vi "Configure Measurement Characteristics (Frequency-Power).vi"(0 "VISA resource name":refnum<visa-resource-name>, 1 "Trace 1 Format Settings":T2={"Frequency Format (1: Hz)"=enum."Hz", "Sensitivity Aperture (1 %)"=1.0, "Frequency Reference (0 Hz)"=0.0} {"Frequency Reference (0 Hz)" format="%^#_9g"; "Sensitivity Aperture (1 %)" format="%^#_9g"}, 5 "Frequency Band (1: High)":u16(ring)=1 items=["Low (10E6 to 1.5E9 Hz)", "High (250E6 to 7E9 Hz)", "Band 3 (3E9 to 10E9 Hz)", "Band 4 (9E9 to 26.5E9 Hz)"], 7 "Enable Carrier Search (Disable)":bool, 9 "Manual Nominal Frequency (3E9 Hz)":dbl=3000000000.0 format="%^#_9g", 11 "error in (no error)":errorcluster, 12 "Trace 4 Format Settings":T1={"Frequency Format (2: Hz/V)"=enum."Hz/V", "Sensitivity Aperture (1 %)"=1.0, "Frequency Reference (0 Hz)"=0.0} {"Frequency Reference (0 Hz)" format="%^#_9g"; "Sensitivity Aperture (1 %)" format="%^#_9g"}) -> (4 "VISA resource name out":refnum<visa-resource-name>, 15 "error out":errorcluster)   [LabVIEW 2011, in "Agilent E5052X.lvlib"]
doc: "Configures initial settings for Frequency/Power measurement. \n\n<b>Note: </b>\n\n1) This VI must be called first before calling \"Configure Measurement(Freq-Power)\" VI.\n\n2) Only Trace 1 and 4 format settings can be changed. Trace 2 and 3 are constantly set for Power and Current respectively."
uses:
  Agilent E5052X.lvlib
panel:
  # "Input Frequency Setting"
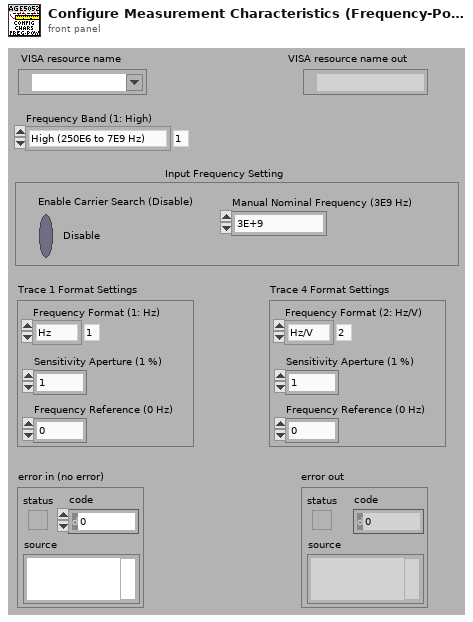
[diagram p1: front panel]
types:
  T1 = cluster{"Frequency Format (2: Hz/V)":enum16{"DHz", "Hz", "Hz/V", "Percent", "ppm"}, "Sensitivity Aperture (1 %)":dbl, "Frequency Reference (0 Hz)":dbl}
  T2 = cluster{"Frequency Format (1: Hz)":enum16{"DHz", "Hz", "Hz/V", "Percent", "ppm"}, "Sensitivity Aperture (1 %)":dbl, "Frequency Reference (0 Hz)":dbl}
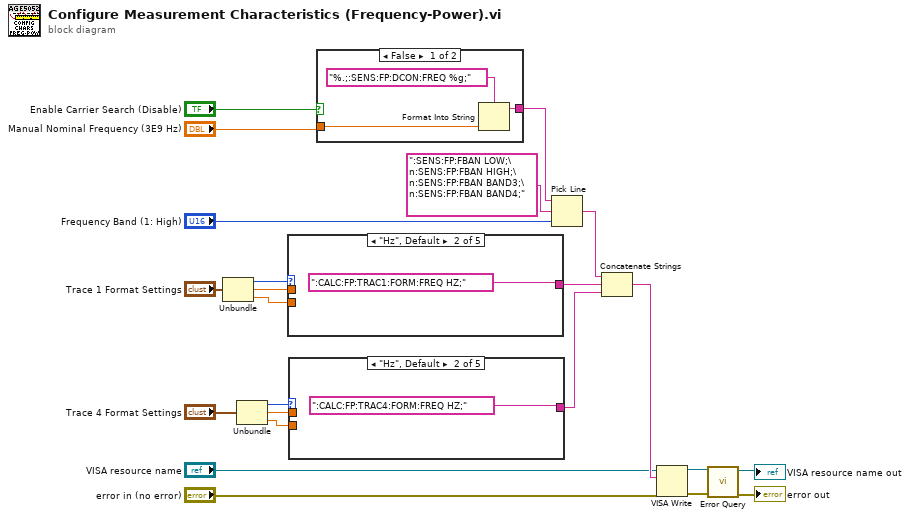
[diagram p0: block diagram]
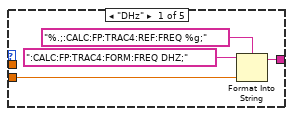
[diagram p2: hidden frame]
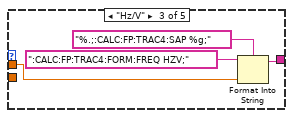
[diagram p3: hidden frame]
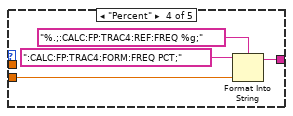
[diagram p4: hidden frame]
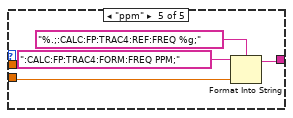
[diagram p5: hidden frame]
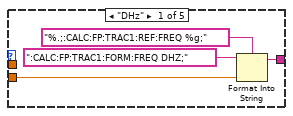
[diagram p6: hidden frame]
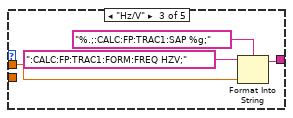
[diagram p7: hidden frame]
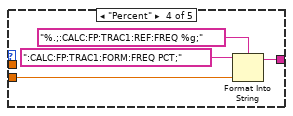
[diagram p8: hidden frame]
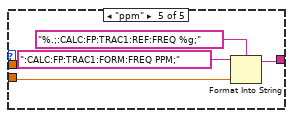
[diagram p9: hidden frame]
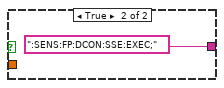
[diagram p10: hidden frame]
diagram:
  n1 = Unbundle("Trace 1 Format Settings") -> ("Frequency Format (1: Hz)"=w19:enum16{"DHz", "Hz", "Hz/V", "Percent", "ppm"}, "Sensitivity Aperture (1 %)"=w17:dbl, "Frequency Reference (0 Hz)"=w18:dbl)
  n2 = Unbundle("Trace 4 Format Settings") -> ("Frequency Format (2: Hz/V)"=w15:enum16{"DHz", "Hz", "Hz/V", "Percent", "ppm"}, "Sensitivity Aperture (1 %)"=w14:dbl, "Frequency Reference (0 Hz)"=w16:dbl)
  n3 = case shown="\"Hz\", Default" w19 {
    tunnel: w18 -> [w26 _ _ w34 w38]
    tunnel: w17 -> [_ _ w30 _ _]
    tunnel: [w24 ":CALC:FP:TRAC1:FORM:FREQ HZ;" w29 w33 w37] -> w13
    frame "DHz" {
      n4 = Format Into String(format string="%.;:CALC:FP:TRAC1:REF:FREQ %g;", initial string=":CALC:FP:TRAC1:FORM:FREQ DHZ;", w26) -> (resulting string=w24:string)  [unwired: 1 in, 1 out]
    }
    frame "Hz", Default {
    }
    frame "Hz/V" {
      n5 = Format Into String(format string="%.;:CALC:FP:TRAC1:SAP %g;", initial string=":CALC:FP:TRAC1:FORM:FREQ HZV;", w30) -> (resulting string=w29:string)  [unwired: 1 in, 1 out]
    }
    frame "Percent" {
      n6 = Format Into String(format string="%.;:CALC:FP:TRAC1:REF:FREQ %g;", initial string=":CALC:FP:TRAC1:FORM:FREQ PCT;", w34) -> (resulting string=w33:string)  [unwired: 1 in, 1 out]
    }
    frame "ppm" {
      n7 = Format Into String(format string="%.;:CALC:FP:TRAC1:REF:FREQ %g;", initial string=":CALC:FP:TRAC1:FORM:FREQ PPM;", w38) -> (resulting string=w37:string)  [unwired: 1 in, 1 out]
    }
  }
  n8 = case shown="\"Hz\", Default" w15 {
    tunnel: w16 -> [w43 _ _ w51 w55]
    tunnel: w14 -> [_ _ w47 _ _]
    tunnel: [w41 ":CALC:FP:TRAC4:FORM:FREQ HZ;" w46 w50 w54] -> w12
    frame "DHz" {
      n9 = Format Into String(format string="%.;:CALC:FP:TRAC4:REF:FREQ %g;", initial string=":CALC:FP:TRAC4:FORM:FREQ DHZ;", w43) -> (resulting string=w41:string)  [unwired: 1 in, 1 out]
    }
    frame "Hz", Default {
    }
    frame "Hz/V" {
      n10 = Format Into String(format string="%.;:CALC:FP:TRAC4:SAP %g;", initial string=":CALC:FP:TRAC4:FORM:FREQ HZV;", w47) -> (resulting string=w46:string)  [unwired: 1 in, 1 out]
    }
    frame "Percent" {
      n11 = Format Into String(format string="%.;:CALC:FP:TRAC4:REF:FREQ %g;", initial string=":CALC:FP:TRAC4:FORM:FREQ PCT;", w51) -> (resulting string=w50:string)  [unwired: 1 in, 1 out]
    }
    frame "ppm" {
      n12 = Format Into String(format string="%.;:CALC:FP:TRAC4:REF:FREQ %g;", initial string=":CALC:FP:TRAC4:FORM:FREQ PPM;", w55) -> (resulting string=w54:string)  [unwired: 1 in, 1 out]
    }
  }
  n13 = case shown="False" "Enable Carrier Search (Disable)" {
    tunnel: "Manual Nominal Frequency (3E9 Hz)" -> [w60 _]
    tunnel: [w58 ":SENS:FP:DCON:SSE:EXEC;" ("write buffer")] -> w3
    frame False {
      n14 = Format Into String(format string="%.;:SENS:FP:DCON:FREQ %g;", w60) -> (resulting string=w58:string)  [unwired: 2 in, 1 out]
    }
    frame True {
    }
  }
  n15 = Pick Line(string ("")=w3, multi-line string=":SENS:FP:FBAN LOW;\n:SENS:FP:FBAN HIGH;\n:SENS:FP:FBAN BAND3;\n:SENS:FP:FBAN BAND4;", line index="Frequency Band (1: High)") -> (output string=w1:string)
  n16 = Concatenate Strings(w1, w13, w12) -> (w11:string)
  n17 = VISA Write(VISA resource name="VISA resource name", write buffer=w11, error in (no error)="error in (no error)") -> (VISA resource name out=w10:refnum<visa-resource-name>, error out=w9:errorcluster)  [unwired: 1 out]
  n18 = call "Error Query.vi"("error in (no error)"=w9, "VISA resource name"=w10) -> ("error out"=→"error out":errorcluster, "VISA resource name out"=→"VISA resource name out":refnum<visa-resource-name>)  [unwired: 6 in, 2 out]
